vi "WPI_AccelerometerADXL345_SPI_Get.vi"(8 "error in":errorcluster, 11 "AccelerometerDevRef":T2={"DevStatus"={"status"=FALSE, "code"=0, "source"=""}, "Scaling"={"Gain (VoltsPerG)"=0.0, "Center Voltage"=0.0}, "Analog Channels"={"X-Axis"=enum."Invalid", "Y-Axis"=enum."Invalid", "Z-Axis"=enum."Invalid"}, "I2C Bus"=enum."Invalid", "SPI Bus"=enum."Invalid", "Accel Range"=0, "ADXL Axes"={"X-Axis"=FALSE, "Y-Axis"=FALSE, "Z-Axis"=FALSE}, "Handle"=0, "Device Address"=0, "Accel Type"=enum."Analog"} {"Device Address" format="%.0x"; "Accel Range" items=["+/- 2 g", "+/- 4 g", "+/- 8 g", "+/- 16 g"]}) -> (0 "error out":errorcluster, 2 "Accelerations":T1, 3 "AccelerometerDevRef":T2={"DevStatus"={"status"=FALSE, "code"=0, "source"=""}, "Scaling"={"Gain (VoltsPerG)"=0.0, "Center Voltage"=0.0}, "Analog Channels"={"X-Axis"=enum."Invalid", "Y-Axis"=enum."Invalid", "Z-Axis"=enum."Invalid"}, "I2C Bus"=enum."Invalid", "SPI Bus"=enum."Invalid", "Accel Range"=0, "ADXL Axes"={"X-Axis"=FALSE, "Y-Axis"=FALSE, "Z-Axis"=FALSE}, "Handle"=0, "Device Address"=0, "Accel Type"=enum."Analog"} {"Device Address" format="%.0x"; "Accel Range" items=["+/- 2 g", "+/- 4 g", "+/- 8 g", "+/- 16 g"]})   [LabVIEW 2017]
doc: "Returns the current acceleration of the sensor that you specify.\n\nThis software is licensed. Open the labview\\readme\\WPI Robotics Library Open Source License.txt file for more information."
uses:
  <vilib>/Rock Robotics/WPI/Accelerometer/WPI_AccelerometerDevRef.ctl
  <vilib>/Rock Robotics/WPI/Accelerometer/WPI_AccelerometerScaling.ctl
  <vilib>/Rock Robotics/WPI/Accelerometer/WPI_AccelerometerAnalogChannels.ctl
  <vilib>/Rock Robotics/SystemInterfaces/AI/FPGA_AIChannel.ctl
  <vilib>/Rock Robotics/SystemInterfaces/i2clib/i2c_bus.ctl
  <vilib>/Rock Robotics/SystemInterfaces/spilib/spi_bus.ctl
  <vilib>/Rock Robotics/WPI/Accelerometer/ADXL345 Range.ctl
  <vilib>/Rock Robotics/WPI/Accelerometer/WPI_AccelerometerADXL345 Axes.ctl
  <vilib>/Rock Robotics/WPI/SPI/WPI_SPIDevRef.ctl
panel:
  # "ADXL"
  # "Analog"
  # "ADXL"
  # "Analog"
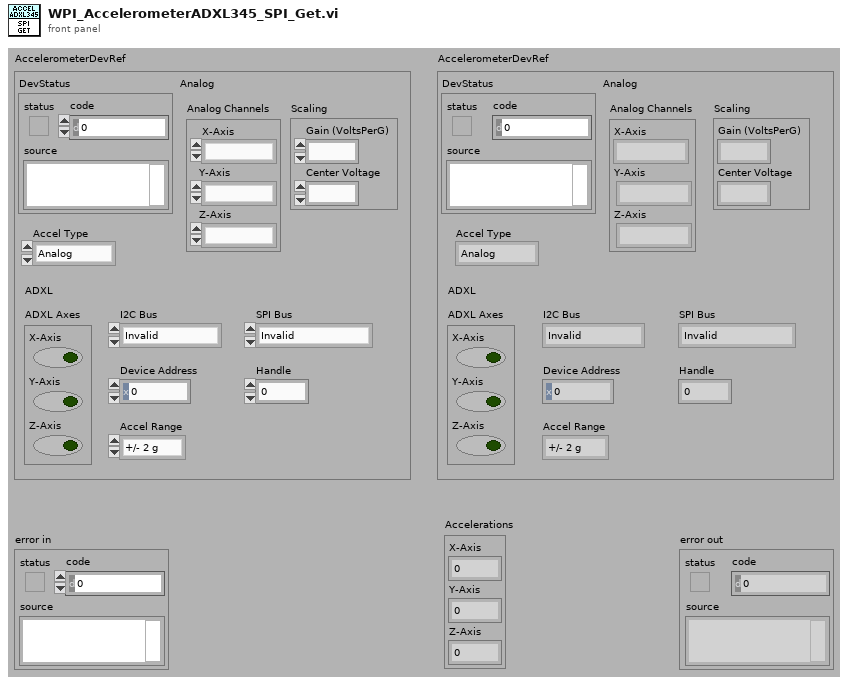
[diagram p1: front panel]
types:
  T1 = cluster{"X-Axis":dbl, "Y-Axis":dbl, "Z-Axis":dbl}
  T2 = typedef "WPI_AccelerometerDevRef.ctl" = cluster{"DevStatus":errorcluster, "Scaling":T3, "Analog Channels":T4, "I2C Bus":T6, "SPI Bus":T7, "Accel Range":T8, "ADXL Axes":T9, "Handle":i32, "Device Address":u8, "Accel Type":enum16{"Analog", "ADXL345 I2C", "ADXL345 SPI", "Internal", "ADXL362 SPI"}}
  T3 = typedef "WPI_AccelerometerScaling.ctl" = cluster{"Gain (VoltsPerG)":dbl, "Center Voltage":dbl}
  T4 = typedef "WPI_AccelerometerAnalogChannels.ctl" = cluster{"X-Axis":T5, "Y-Axis":T5, "Z-Axis":T5}
  T5 = typedef "FPGA_AIChannel.ctl" = enum8{"AI 0", "AI 1", "AI 2", "AI 3", "AI MXP 0", "AI MXP 1", "AI MXP 2", "AI MXP 3", "Invalid"}
  T6 = typedef "i2c_bus.ctl" = enum16{"I2C On-Board", "I2C MXP", "Invalid"}
  T7 = typedef "spi_bus.ctl" = enum16{"SPI On-Board, CS0", "SPI On-Board, CS1", "SPI On-Board, CS2", "SPI On-Board, CS3", "SPI MXP", "Invalid"}
  T8 = typedef "ADXL345 Range.ctl" = u8
  T9 = typedef "WPI_AccelerometerADXL345 Axes.ctl" = cluster{"X-Axis":bool, "Y-Axis":bool, "Z-Axis":bool}
  T10 = typedef "WPI_SPIDevRef.ctl" = cluster{"DevStatus":errorcluster, "Handle":i32, "SPI Bus":T7}
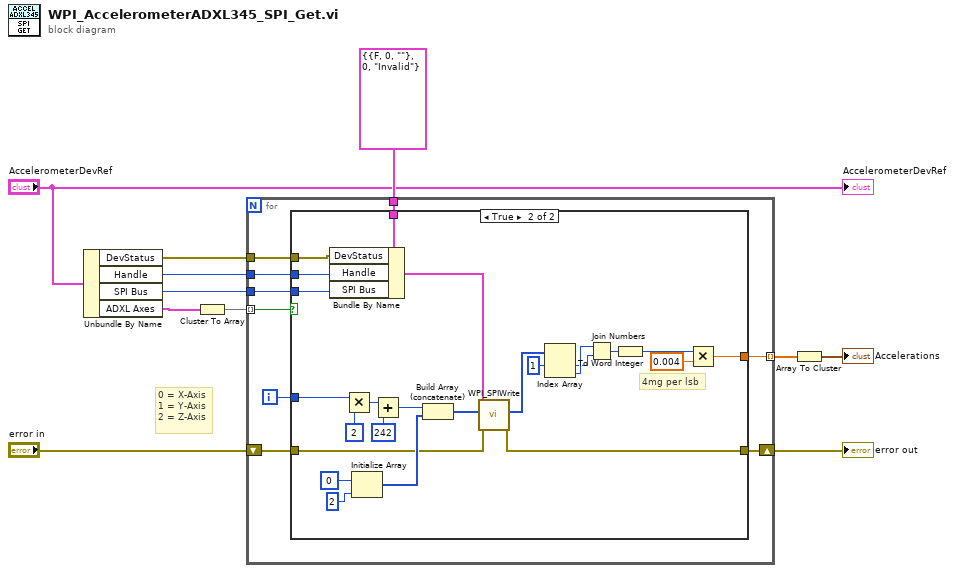
[diagram p0: block diagram]
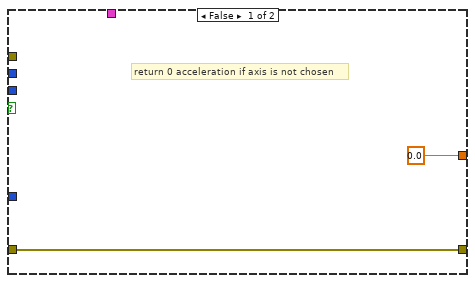
[diagram p2: hidden frame]
diagram:
  # "0 = X-Axis\n1 = Y-Axis\n2 = Z-Axis"
  n1 = Unbundle By Name("AccelerometerDevRef") -> ("DevStatus"=w8:errorcluster, "Handle"=w9:i32, "SPI Bus"=w6:T7, "ADXL Axes"=w4:T9)
  n2 = Cluster To Array(cluster=w4) -> (array=w3:bool[])
  n3 = for {
    shift-right: [w20] -> w11
    shift-left: "error in" -> [w19]
    tunnel: T10 {"DevStatus"={"status"=FALSE, "code"=0, "source"=""}, "Handle"=0, "SPI Bus"=enum."Invalid"} ("SPIDevRef") -> [w18]
    tunnel: w9 -> [w17]
    tunnel: w8 -> [w16]
    tunnel: w6 -> [w15]
    tunnel: [w14] -> w5 mode=indexing
    tunnel: w3 -> [w13] mode=indexing
    i -> [w12]
    n4 = case shown="True" w13 {
      tunnel: [w22 w23] -> w20
      tunnel: w19 -> [w22 w24]
      tunnel: w18 -> [_ w46]
      tunnel: w17 -> [_ w45]
      tunnel: w16 -> [_ w44]
      tunnel: w15 -> [_ w43]
      tunnel: [0.0 ("Voltage") w25] -> w14
      tunnel: w12 -> [_ w27]
      frame False {
        # "return 0 acceleration if axis is not chosen"
      }
      frame True {
        # "4mg per lsb"
        n5 = Bundle By Name(cluster=w46, "DevStatus"=w44, "Handle"=w45, "SPI Bus"=w43) -> (w26:T10)
        n6 = Multiply(x=w27, y=u32 2 ("Data To Send")) -> (x*y=w42:u32)
        n7 = Initialize Array(u32 0 ("Data To Send"), 2 ("dimension size")) -> (w36:u32[])
        n8 = Add(x=w42, y=u32 242 ("Data To Send")) -> (x+y=w35:u32)
        n9 = Build Array (concatenate)(w35, w36) -> (w34:u32[])
        n10 = call <vilib>:"WPI_SPIWrite.vi"("error in (no error)"=w24, "Data To Send"=w34, "SPIDevRef"=w26) -> ("error out"=w23:errorcluster, "Received Data"=w33:u8[])  [unwired: 7 out]
        n11 = Index Array(array=w33, index #1=1 ("index")) -> (element #1=w28:u8, element #2=w29:u8)  [unwired: 1 in]
        n12 = Join Numbers(hi=w29, lo=w28) -> ((hi.lo)=w31:u16)
        n13 = To Word Integer(number=w31) -> (16bit integer=w30:i16)
        n14 = Multiply(x=w30, y=0.004) -> (x*y=w25:dbl)
      }
    }
  }
  "error out" <- w11
  n15 = Array To Cluster(array=w5) -> (cluster=→"Accelerations":cluster{"[0]":dbl, "[1]":dbl, "[2]":dbl})
  "AccelerometerDevRef" <- "AccelerometerDevRef"
